vi "connect.vi"(8 "error in (no error)":errorcluster, 11 "StimulatorAK101022TCP in":refnum<class "StimulatorAK101022TCP.lvclass">) -> (0 "error out":errorcluster, 2 "connected":bool, 3 "StimulatorAK101022TCP out":refnum<class "StimulatorAK101022TCP.lvclass">)   [LabVIEW 2010, in "StimulatorAK101022TCP.lvclass"]
uses:
  StimulatorAK101022TCP.lvclass
  StimulatorAK101022TCP.lvclass/StimulatorAK101022TCP.ctl
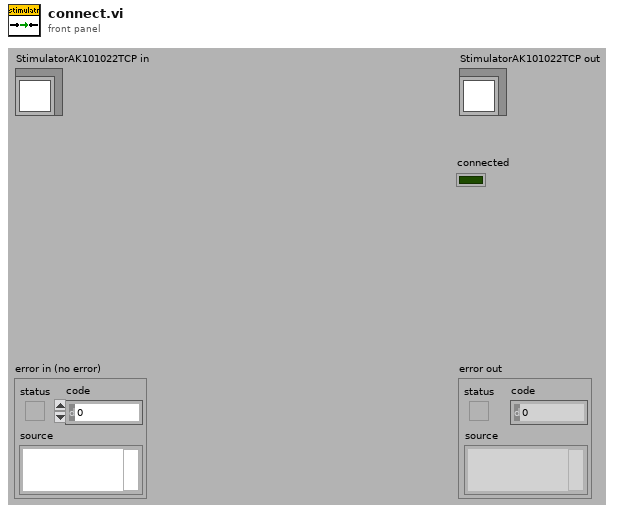
[diagram p1: front panel]
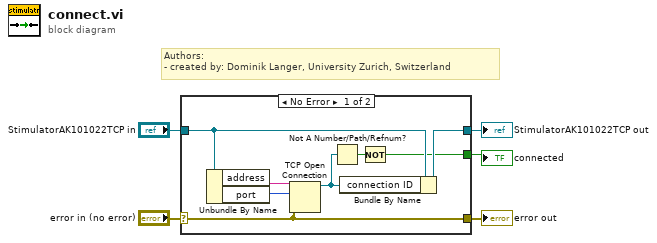
[diagram p0: block diagram]
diagram:
  # "Authors: \n- created by: Dominik Langer, University Zurich, Switzerland"
  n1 = case shown="No Error" "error in (no error)" {
    selector: "error in (no error)" -> [w6 w15]
    tunnel: [w6 w15] -> w4
    tunnel: [w8 w14] -> w2
    tunnel: "StimulatorAK101022TCP in" -> [w9 w14]
    tunnel: [w7 _] -> w1
    frame No Error {
      n2 = Unbundle By Name(w9) -> ("address"=w12:string, "port"=w13:u16)
      n3 = TCP Open Connection(address=w12, remote port or service name=w13, error in (no error)=w6) -> (connection ID=w10:refnum<k5>)  [unwired: 2 in, 1 out]
      n4 = Not A Number/Path/Refnum?(number/path/refnum=w10) -> (NaN/Path/Refnum?=w11:bool)
      n5 = Bundle By Name(cluster=w9, "connection ID"=w10) -> (w8:refnum<class "StimulatorAK101022TCP.lvclass">)
      n6 = Not(x=w11) -> (.not. x?=w7:bool)
    }
    frame Error {
    }
  }
  "error out" <- w4
  "StimulatorAK101022TCP out" <- w2
  "connected" <- w1
